vi "Indent.vi"(11 "MsgSerializer in":refnum<class "MsgSerializer.JSON.lvclass">) -> (3 "MsgSerializer out":refnum<class "MsgSerializer.JSON.lvclass">)   [LabVIEW 2013]
uses:
  MsgSerializer.JSON.lvclass
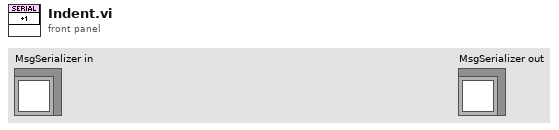
[diagram p1: front panel]
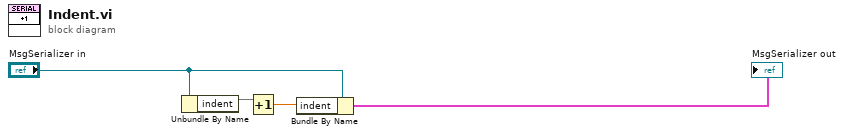
[diagram p0: block diagram]
diagram:
  n1 = Unbundle By Name("MsgSerializer in") -> ("indent"=w4)
  n2 = Increment(x=w4) -> (x+1=w3:dbl)
  n3 = Bundle By Name(cluster="MsgSerializer in", "indent"=w3) -> (→"MsgSerializer out":cluster{})
